vi "GetValuesMatchingXPath.vi"(8 "error in (no error)":errorcluster, 10 "XPath":string, 11 "XML refnum in":refnum<k20>) -> (0 "error out":errorcluster, 2 "Values":string[](array[string]), 3 "XML refnum out":refnum<k20>)   [LabVIEW 2015, in "VeriStandTestUtilities.lvlib"]
uses:
  VeriStandTestUtilities.lvlib
  <resource>/objmgr/DOMUserDefRef.rc
  <vilib>/xml/NI_XML.lvlib
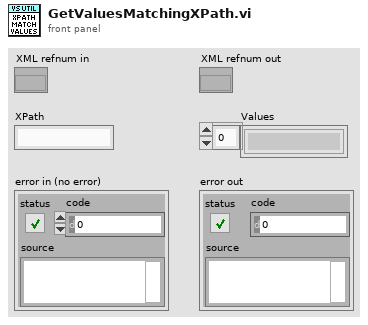
[diagram p1: front panel]
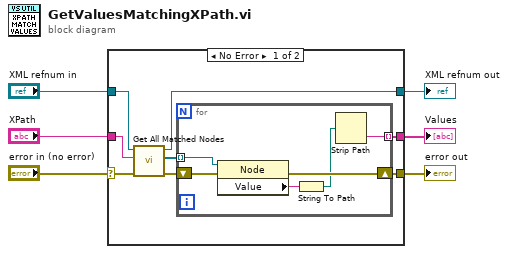
[diagram p0: block diagram]
diagram:
  n1 = case shown="No Error" "error in (no error)" {
    selector: "error in (no error)" -> [w10 w21]
    tunnel: [w14 w21] -> w6
    tunnel: [w13 _] -> w5
    tunnel: "XPath" -> [w12 _]
    tunnel: [w11 w22] -> w3
    tunnel: "XML refnum in" -> [w9 w22]
    frame No Error {
      n2 = call <vilib>:"Get All Matched Nodes.vi"("error in (no error)"=w10, "XPath expression"=w12, "node in"=w9) -> ("error out"=w7:errorcluster, "node result array"=w8:refnum<k20>[], "node out"=w11:refnum<k20>)  [unwired: 6 in]
      n3 = for {
        shift-right: [w19] -> w14
        shift-left: w7 -> [w20]
        tunnel: w8 -> [w18] mode=indexing
        tunnel: [w15] -> w13 mode=indexing
        n4 = property class="Node"(reference=w18, error in=w20) -> (error out=w19:errorcluster, "Value"=w16:string)  [unwired: 1 out]
        n5 = String To Path(string=w16) -> (path=w17:path)
        n6 = Strip Path(path=w17) -> (name=w15:string)  [unwired: 1 out]
      }
    }
    frame Error {
    }
  }
  "error out" <- w6
  "Values" <- w5
  "XML refnum out" <- w3
